vi "7Segment_24_Display.vi"(2 "24Time":u32) -> ()   [LabVIEW 2020]
panel:
  out "7Segment1sec":T1
  out "7Segment10sec":T1
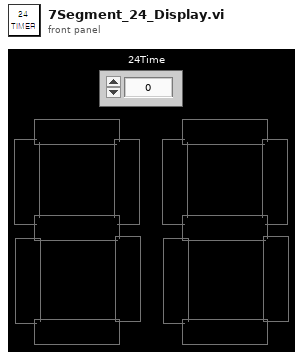
[diagram p1: front panel]
types:
  T1 = cluster{"Led 4":bool, "Led":bool, "Led 3":bool, "Led 2":bool, "Led 5":bool, "Led 6":bool, "Led 7":bool}
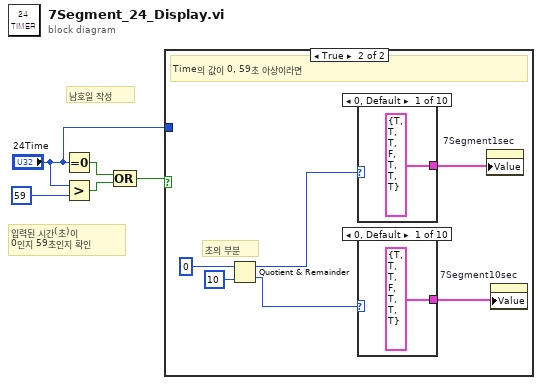
[diagram p0: block diagram]
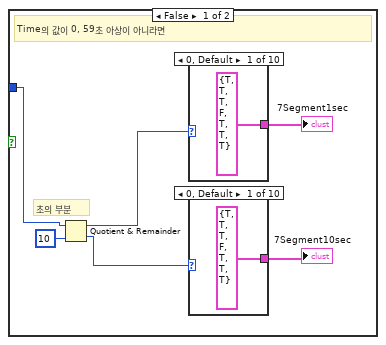
[diagram p2: hidden frame]
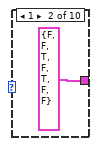
[diagram p3: hidden frame]
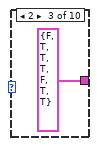
[diagram p4: hidden frame]
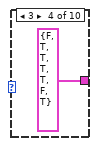
[diagram p5: hidden frame]
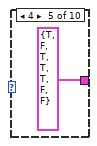
[diagram p6: hidden frame]
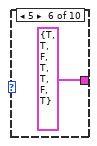
[diagram p7: hidden frame]
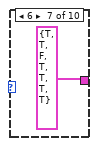
[diagram p8: hidden frame]
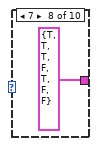
[diagram p9: hidden frame]
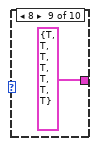
[diagram p10: hidden frame]
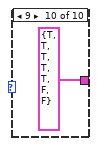
[diagram p11: hidden frame]
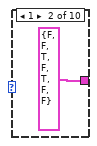
[diagram p12: hidden frame]
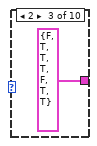
[diagram p13: hidden frame]
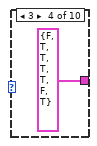
[diagram p14: hidden frame]
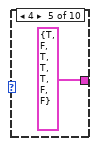
[diagram p15: hidden frame]
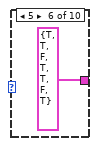
[diagram p16: hidden frame]
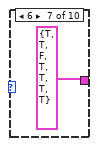
[diagram p17: hidden frame]
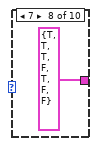
[diagram p18: hidden frame]
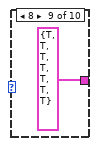
[diagram p19: hidden frame]
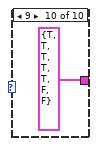
[diagram p20: hidden frame]
diagram:
  # "입력된 시간(초)이\n0인지 59초인지 확인"
  # "남호일 작성"
  n1 = Equal To 0?(x="24Time") -> (x = 0?=w4:bool)
  n2 = Greater?(x="24Time", y=59) -> (0:w3:bool)
  n3 = Compound Arithmetic op=OR(w4, w3) -> (w2:bool)
  n4 = case shown="True" w2 {
    tunnel: "24Time" -> [w6 _]
    frame False {
      # "초의 부분"
      # "Time의 값이 0, 59초 아상이 아니라면"
      n5 = Quotient & Remainder(x=w6, y=u16 10) -> (x-y*floor(x/y)=w9:u32, floor(x/y)=w10:u32)
      n6 = case shown="0, Default" w9 {
        tunnel: [T1 {"Led 4"=TRUE, "Led"=TRUE, "Led 3"=TRUE, "Led 2"=FALSE, "Led 5"=TRUE, "Led 6"=TRUE, "Led 7"=TRUE} ("7Segment10min") T1 {"Led 4"=FALSE, "Led"=FALSE, "Led 3"=TRUE, "Led 2"=FALSE, "Led 5"=TRUE, "Led 6"=FALSE, "Led 7"=FALSE} ("7Segment10min") T1 {"Led 4"=FALSE, "Led"=TRUE, "Led 3"=TRUE, "Led 2"=TRUE, "Led 5"=FALSE, "Led 6"=TRUE, "Led 7"=TRUE} ("7Segment10min") T1 {"Led 4"=FALSE, "Led"=TRUE, "Led 3"=TRUE, "Led 2"=TRUE, "Led 5"=TRUE, "Led 6"=FALSE, "Led 7"=TRUE} ("7Segment10min") T1 {"Led 4"=TRUE, "Led"=FALSE, "Led 3"=TRUE, "Led 2"=TRUE, "Led 5"=TRUE, "Led 6"=FALSE, "Led 7"=FALSE} ("7Segment10min") T1 {"Led 4"=TRUE, "Led"=TRUE, "Led 3"=FALSE, "Led 2"=TRUE, "Led 5"=TRUE, "Led 6"=FALSE, "Led 7"=TRUE} ("7Segment10min") T1 {"Led 4"=TRUE, "Led"=TRUE, "Led 3"=FALSE, "Led 2"=TRUE, "Led 5"=TRUE, "Led 6"=TRUE, "Led 7"=TRUE} ("7Segment10min") T1 {"Led 4"=TRUE, "Led"=TRUE, "Led 3"=TRUE, "Led 2"=FALSE, "Led 5"=TRUE, "Led 6"=FALSE, "Led 7"=FALSE} ("7Segment10min") T1 {"Led 4"=TRUE, "Led"=TRUE, "Led 3"=TRUE, "Led 2"=TRUE, "Led 5"=TRUE, "Led 6"=TRUE, "Led 7"=TRUE} ("7Segment10min") T1 {"Led 4"=TRUE, "Led"=TRUE, "Led 3"=TRUE, "Led 2"=TRUE, "Led 5"=TRUE, "Led 6"=FALSE, "Led 7"=FALSE} ("7Segment10min")] -> w7
        frame 0, Default {
        }
        frame 1 {
        }
        frame 2 {
        }
        frame 3 {
        }
        frame 4 {
        }
        frame 5 {
        }
        frame 6 {
        }
        frame 7 {
        }
        frame 8 {
        }
        frame 9 {
        }
      }
      "7Segment1sec" <- w7
      n7 = case shown="0, Default" w10 {
        tunnel: [T1 {"Led 4"=TRUE, "Led"=TRUE, "Led 3"=TRUE, "Led 2"=FALSE, "Led 5"=TRUE, "Led 6"=TRUE, "Led 7"=TRUE} ("7Segment10min") T1 {"Led 4"=FALSE, "Led"=FALSE, "Led 3"=TRUE, "Led 2"=FALSE, "Led 5"=TRUE, "Led 6"=FALSE, "Led 7"=FALSE} ("7Segment10min") T1 {"Led 4"=FALSE, "Led"=TRUE, "Led 3"=TRUE, "Led 2"=TRUE, "Led 5"=FALSE, "Led 6"=TRUE, "Led 7"=TRUE} ("7Segment10min") T1 {"Led 4"=FALSE, "Led"=TRUE, "Led 3"=TRUE, "Led 2"=TRUE, "Led 5"=TRUE, "Led 6"=FALSE, "Led 7"=TRUE} ("7Segment10min") T1 {"Led 4"=TRUE, "Led"=FALSE, "Led 3"=TRUE, "Led 2"=TRUE, "Led 5"=TRUE, "Led 6"=FALSE, "Led 7"=FALSE} ("7Segment10min") T1 {"Led 4"=TRUE, "Led"=TRUE, "Led 3"=FALSE, "Led 2"=TRUE, "Led 5"=TRUE, "Led 6"=FALSE, "Led 7"=TRUE} ("7Segment10min") T1 {"Led 4"=TRUE, "Led"=TRUE, "Led 3"=FALSE, "Led 2"=TRUE, "Led 5"=TRUE, "Led 6"=TRUE, "Led 7"=TRUE} ("7Segment10min") T1 {"Led 4"=TRUE, "Led"=TRUE, "Led 3"=TRUE, "Led 2"=FALSE, "Led 5"=TRUE, "Led 6"=FALSE, "Led 7"=FALSE} ("7Segment10min") T1 {"Led 4"=TRUE, "Led"=TRUE, "Led 3"=TRUE, "Led 2"=TRUE, "Led 5"=TRUE, "Led 6"=TRUE, "Led 7"=TRUE} ("7Segment10min") T1 {"Led 4"=TRUE, "Led"=TRUE, "Led 3"=TRUE, "Led 2"=TRUE, "Led 5"=TRUE, "Led 6"=FALSE, "Led 7"=FALSE} ("7Segment10min")] -> w8
        frame 0, Default {
        }
        frame 1 {
        }
        frame 2 {
        }
        frame 3 {
        }
        frame 4 {
        }
        frame 5 {
        }
        frame 6 {
        }
        frame 7 {
        }
        frame 8 {
        }
        frame 9 {
        }
      }
      "7Segment10sec" <- w8
    }
    frame True {
      # "초의 부분"
      # "Time의 값이 0, 59초 아상이라면"
      n8 = Quotient & Remainder(x=u16 0, y=u16 10) -> (x-y*floor(x/y)=w36:u16, floor(x/y)=w37:u16)
      n9 = case shown="0, Default" w36 {
        tunnel: [T1 {"Led 4"=TRUE, "Led"=TRUE, "Led 3"=TRUE, "Led 2"=FALSE, "Led 5"=TRUE, "Led 6"=TRUE, "Led 7"=TRUE} ("7Segment10min") T1 {"Led 4"=FALSE, "Led"=FALSE, "Led 3"=TRUE, "Led 2"=FALSE, "Led 5"=TRUE, "Led 6"=FALSE, "Led 7"=FALSE} ("7Segment10min") T1 {"Led 4"=FALSE, "Led"=TRUE, "Led 3"=TRUE, "Led 2"=TRUE, "Led 5"=FALSE, "Led 6"=TRUE, "Led 7"=TRUE} ("7Segment10min") T1 {"Led 4"=FALSE, "Led"=TRUE, "Led 3"=TRUE, "Led 2"=TRUE, "Led 5"=TRUE, "Led 6"=FALSE, "Led 7"=TRUE} ("7Segment10min") T1 {"Led 4"=TRUE, "Led"=FALSE, "Led 3"=TRUE, "Led 2"=TRUE, "Led 5"=TRUE, "Led 6"=FALSE, "Led 7"=FALSE} ("7Segment10min") T1 {"Led 4"=TRUE, "Led"=TRUE, "Led 3"=FALSE, "Led 2"=TRUE, "Led 5"=TRUE, "Led 6"=FALSE, "Led 7"=TRUE} ("7Segment10min") T1 {"Led 4"=TRUE, "Led"=TRUE, "Led 3"=FALSE, "Led 2"=TRUE, "Led 5"=TRUE, "Led 6"=TRUE, "Led 7"=TRUE} ("7Segment10min") T1 {"Led 4"=TRUE, "Led"=TRUE, "Led 3"=TRUE, "Led 2"=FALSE, "Led 5"=TRUE, "Led 6"=FALSE, "Led 7"=FALSE} ("7Segment10min") T1 {"Led 4"=TRUE, "Led"=TRUE, "Led 3"=TRUE, "Led 2"=TRUE, "Led 5"=TRUE, "Led 6"=TRUE, "Led 7"=TRUE} ("7Segment10min") T1 {"Led 4"=TRUE, "Led"=TRUE, "Led 3"=TRUE, "Led 2"=TRUE, "Led 5"=TRUE, "Led 6"=FALSE, "Led 7"=FALSE} ("7Segment10min")] -> w34
        frame 0, Default {
        }
        frame 1 {
        }
        frame 2 {
        }
        frame 3 {
        }
        frame 4 {
        }
        frame 5 {
        }
        frame 6 {
        }
        frame 7 {
        }
        frame 8 {
        }
        frame 9 {
        }
      }
      n10 = case shown="0, Default" w37 {
        tunnel: [T1 {"Led 4"=TRUE, "Led"=TRUE, "Led 3"=TRUE, "Led 2"=FALSE, "Led 5"=TRUE, "Led 6"=TRUE, "Led 7"=TRUE} ("7Segment10min") T1 {"Led 4"=FALSE, "Led"=FALSE, "Led 3"=TRUE, "Led 2"=FALSE, "Led 5"=TRUE, "Led 6"=FALSE, "Led 7"=FALSE} ("7Segment10min") T1 {"Led 4"=FALSE, "Led"=TRUE, "Led 3"=TRUE, "Led 2"=TRUE, "Led 5"=FALSE, "Led 6"=TRUE, "Led 7"=TRUE} ("7Segment10min") T1 {"Led 4"=FALSE, "Led"=TRUE, "Led 3"=TRUE, "Led 2"=TRUE, "Led 5"=TRUE, "Led 6"=FALSE, "Led 7"=TRUE} ("7Segment10min") T1 {"Led 4"=TRUE, "Led"=FALSE, "Led 3"=TRUE, "Led 2"=TRUE, "Led 5"=TRUE, "Led 6"=FALSE, "Led 7"=FALSE} ("7Segment10min") T1 {"Led 4"=TRUE, "Led"=TRUE, "Led 3"=FALSE, "Led 2"=TRUE, "Led 5"=TRUE, "Led 6"=FALSE, "Led 7"=TRUE} ("7Segment10min") T1 {"Led 4"=TRUE, "Led"=TRUE, "Led 3"=FALSE, "Led 2"=TRUE, "Led 5"=TRUE, "Led 6"=TRUE, "Led 7"=TRUE} ("7Segment10min") T1 {"Led 4"=TRUE, "Led"=TRUE, "Led 3"=TRUE, "Led 2"=FALSE, "Led 5"=TRUE, "Led 6"=FALSE, "Led 7"=FALSE} ("7Segment10min") T1 {"Led 4"=TRUE, "Led"=TRUE, "Led 3"=TRUE, "Led 2"=TRUE, "Led 5"=TRUE, "Led 6"=TRUE, "Led 7"=TRUE} ("7Segment10min") T1 {"Led 4"=TRUE, "Led"=TRUE, "Led 3"=TRUE, "Led 2"=TRUE, "Led 5"=TRUE, "Led 6"=FALSE, "Led 7"=FALSE} ("7Segment10min")] -> w33
        frame 0, Default {
        }
        frame 1 {
        }
        frame 2 {
        }
        frame 3 {
        }
        frame 4 {
        }
        frame 5 {
        }
        frame 6 {
        }
        frame 7 {
        }
        frame 8 {
        }
        frame 9 {
        }
      }
      n11 = property on="7Segment1sec" class="Clust (strict)"("Value"=w34) -> ()  [unwired: 2 in, 2 out]
      n12 = property on="7Segment10sec" class="Clust (strict)"("Value"=w33) -> ()  [unwired: 2 in, 2 out]
    }
  }
